vi "Read Mode.vi"(8 "error in (no error)":errorcluster, 11 "DAQ Class in":refnum<class "DAQ Class.lvclass">) -> (0 "error out":errorcluster, 2 "Mode":T1, 3 "DAQ Class out":refnum<class "DAQ Class.lvclass">)   [LabVIEW 2015, in "DAQ Class.lvclass"]
uses:
  DAQ Class.lvclass
  DAQ Modes.ctl
  DAQ Class.lvclass/DAQ Class.ctl
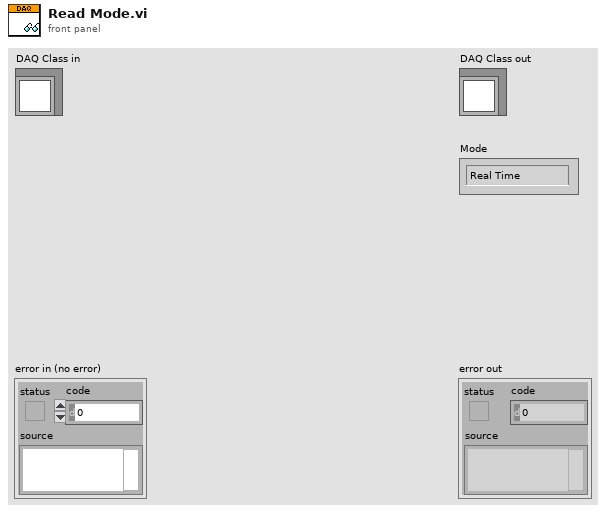
[diagram p1: front panel]
types:
  T1 = typedef "DAQ Class.lvclass/DAQ Modes.ctl" = enum16{"Real Time", "Save Data"}
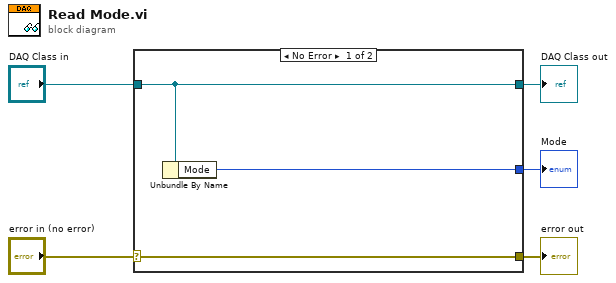
[diagram p0: block diagram]
diagram:
  n1 = case shown="No Error" "error in (no error)" {
    selector: "error in (no error)" -> [w8 w9]
    tunnel: [w8 w9] -> w4
    tunnel: [w7 w10] -> w2
    tunnel: "DAQ Class in" -> [w7 w10]
    tunnel: [w6 _] -> w1
    frame No Error {
      n2 = Unbundle By Name(w7) -> ("Mode"=w6:T1)
    }
    frame Error {
    }
  }
  "error out" <- w4
  "DAQ Class out" <- w2
  "Mode" <- w1
